vi "Elmin Mejia Prueba 1.vi"() -> ()   [LabVIEW 2011]
panel:
  out "601-1000 LLENADO":bool
  out "301-600 MEDIO":bool
  out "1-300 VACIO":bool
  out "Tanque":i32(slide) scale=1.0..1000.0
  # "EL PROGRAMA DEBERA DE LLENAR EL TANQUE\nLA BOMBA GENERA DE 1-50 GALONES, LOS CUALES\nSE SUMAN Y ESTA SUMA SE REPRESENTA POR EL \nTANQUE.  \nDEBERA DE IR ENCENDIENDO LOS LED DE ACUERDO\nAL VOLUMEN DE AGUA DEL TANQUE.\nCUANDO ESTE SE LLNE SE DETIENE EL PROGRAMA.\nNOTA: LLENADO SE ENTIENDE CUANDO LA SUMA\nES IGUAL A 1000 O MAYOR."
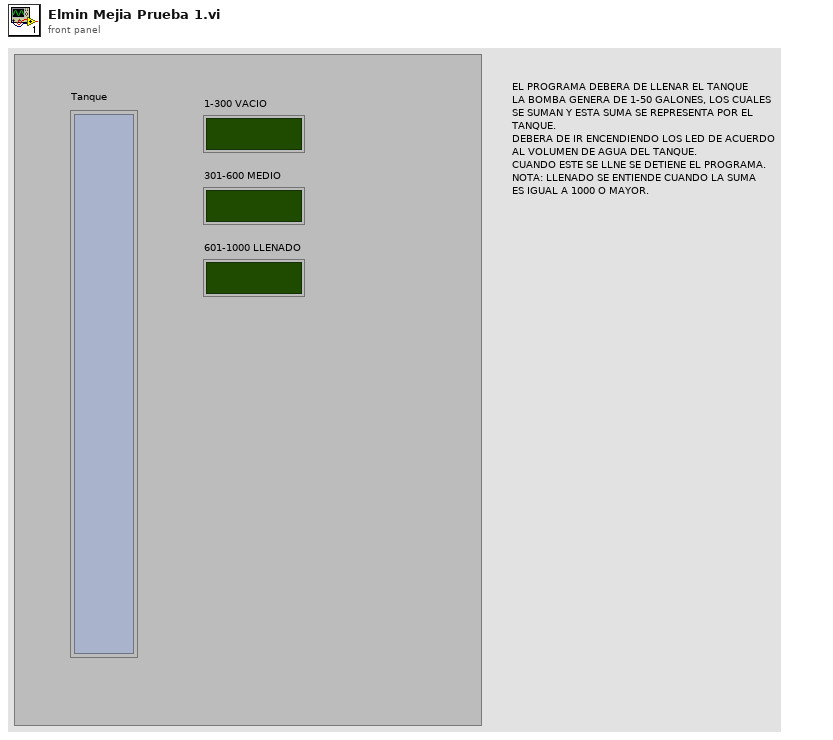
[diagram p1: front panel]
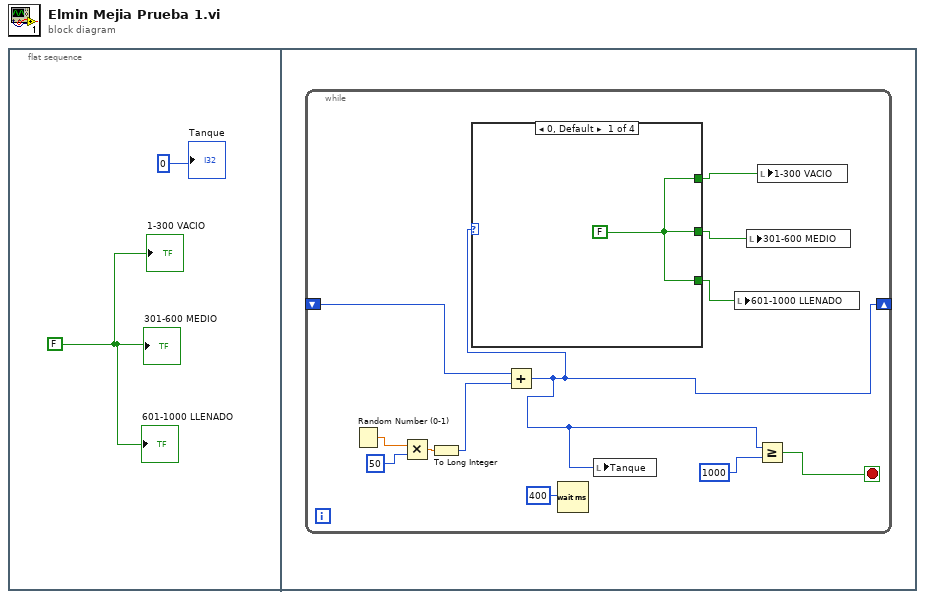
[diagram p0: block diagram]
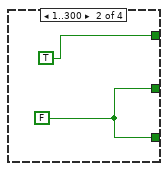
[diagram p2: hidden frame]
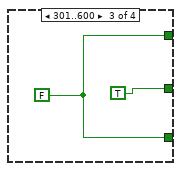
[diagram p3: hidden frame]
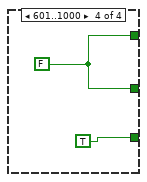
[diagram p4: hidden frame]
diagram:
  n1 = flat-sequence {
    frame #0 {
      w1 = FALSE
      "Tanque" <- 0
      "1-300 VACIO" <- w1
      "301-600 MEDIO" <- w1
      "601-1000 LLENADO" <- w1
    }
    frame #1 {
      n2 = while {
        shift-right: [w4] -> _
        shift-left: _ -> [w12]
        stop <- w14 stop-if-true
        n3 = Random Number (0-1)() -> (number: 0 to 1=w8:dbl)
        n4 = Multiply(x=w8, y=50) -> (x*y=w6:dbl)
        n5 = To Long Integer(number=w6) -> (32bit integer=w5:i32)
        n6 = Add(x=w12, y=w5) -> (x+y=w4:i32)
        n7 = case shown="0, Default" w4 {
          tunnel: [w15 TRUE w18 w20] -> w11
          tunnel: [w15 w16 TRUE w20] -> w10
          tunnel: [w15 w16 w18 TRUE] -> w9
          frame 0, Default {
            w15 = FALSE
          }
          frame 1..300 {
            w16 = FALSE
          }
          frame 301..600 {
            w18 = FALSE
          }
          frame 601..1000 {
            w20 = FALSE
          }
        }
        n8 = Wait (ms)(milliseconds to wait=400) -> ()  [unwired: 1 out]
        n9 = local write "Tanque"(w4) -> ()
        n10 = local write "601-1000 LLENADO"(w9) -> ()
        n11 = local write "301-600 MEDIO"(w10) -> ()
        n12 = Greater Or Equal?(x=w4, y=1000) -> (x >= y?=w14:bool)
        n13 = local write "1-300 VACIO"(w11) -> ()
      }
    }
  }
